vi "Initialize.vi"(8 "error in (no error)":errorcluster, 11 "INI Path":path) -> (0 "error out":errorcluster, 3 "connection ID":refnum<k16>)   [LabVIEW 2009, in "UDPComm.lvlib"]
uses:
  UDPComm.lvlib
  <vilib>/Utility/config.llb/Read Key (I32).vi
  <vilib>/Utility/config.llb/NI_LVConfig.lvlib
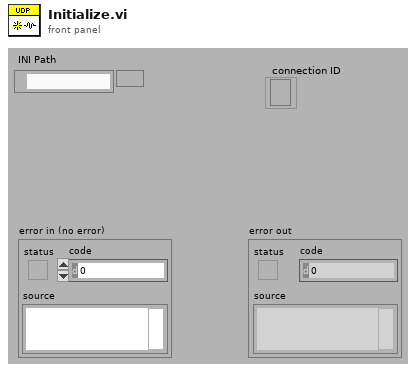
[diagram p1: front panel]
types:
  T1 = typedef "NI_LVConfig.lvlib/Config Data RefNum.ctl" = refnum<k1>
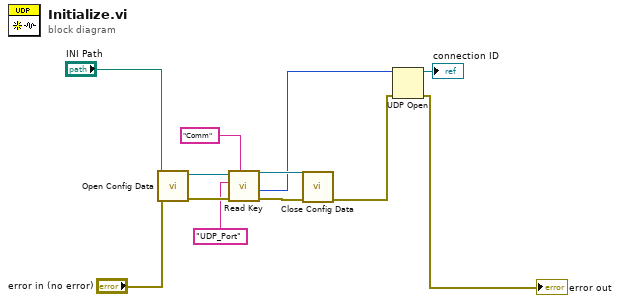
[diagram p0: block diagram]
diagram:
  n1 = call <vilib>:"Open Config Data.vi"("error in (no error)"="error in (no error)", "configuration file path"="INI Path") -> ("error out"=w11:errorcluster, "refnum"=w12:T1)  [unwired: 7 in, 1 out]
  n2 = call-poly <vilib>:"Read Key.vi"("section"="Comm", "error in (no error)"=w11, "key"="UDP_Port", "refnum"=w12) -> ("error out"=w7:errorcluster, "value"=w4:i32, "refnum out"=w8:T1)  [unwired: 4 in, 1 out]
  n3 = call <vilib>:"Close Config Data.vi"("error in (no error)"=w7, "refnum"=w8) -> ("error out"=w2:errorcluster)  [unwired: 8 in, 1 out]
  n4 = UDP Open(8:w2, 11:w4) -> (port=→"connection ID":refnum<k16>, 0:→"error out":errorcluster)  [unwired: 3 in, 1 out]
